vi "Scan Engine-Single Frame.vi"(7 "Channel":u32(ring)=1 items=["A"=1, "B"=2, "A + B"=3, "C"=4, "A + C"=5, "A + B"=6, "D"=8, "A + D"=9, "B + D"=10, "C + D"=12, "A + B + C + D"=15], 8 "Error in":errorcluster, 10 "Scan Status in":T1) -> (0 "Error Out":errorcluster, 2 "Buffer":u16[](array[numeric]), 3 "FFT Buffer":sgl[](array[numeric]))   [LabVIEW 2018]
uses:
  Controls/scan status.ctl
  Hardware Mfg/AlazarTech SDK/Controls/Alazar Engine Actions.ctl
  Controls/FGV Actions.ctl
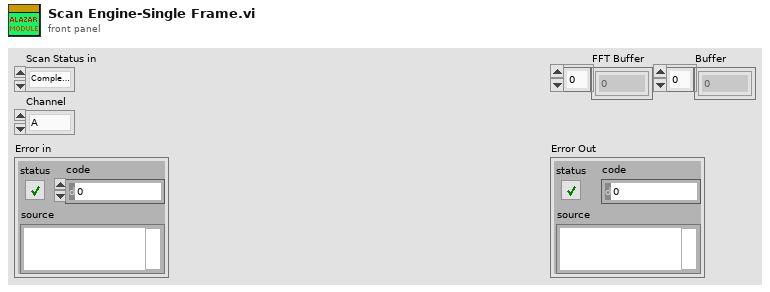
[diagram p1: front panel]
types:
  T1 = typedef "scan status.ctl" = enum16{"Complete Scan(ThorOCT)", "Complete Scan(PSOCT)", "Start(ThorOCT Spatial)", "Start(ThorOCT Spectral)", "Start(GPU FFT)", "Start(Alazar FFT)", "Scan(ThorOCT Spatial)", "Scan(ThorOCT Spectral)", "Scan(GPU FFT)", "Scan(Alazar FFT)", "Finish Scan(ThorOCT)", "Finish Scan(PSOCT)"}
  T2 = typedef "Alazar Engine Actions.ctl" = enum16{"Init", "Config Clock", "Config Ch", "Config Trig", "Config Non-FFT Acq.", "Non-FFT Acquire", "start acquire", "Config Acq.", "Acquire", "UnInit"}
  T3 = typedef "FGV Actions.ctl" = enum16{"Init", "Set", "Get", "Clear"}
  T4 = enum16{"Configure channels", "Write Scan Pattern", "Start Galvo Task", "Is Task Done?", "Stop Galvo", "Uninit", "Init: Calc scan pattern"}
  T5 = typedef "System Parameters.ctl" = cluster{"Optical Parameters":T6, "Vibratome":T7, "Table Stages":T8, "Imaging Parameter":T11, "Galvo HW Parameters":cluster{"Analog Out Channel":tag, "Min Voltage":dbl, "Max Voltage":dbl, "Pixel Clock Source":tag, "Sample Rate":dbl, "Line Clock Out Ch":tag}, "Alazar parameters":T13, "Mosaic Paramter":cluster{"X Axis":cluster{"Start [mm]":dbl, "Steps [pts]":dbl, "End [mm]":dbl}, "Y Axis":cluster{"Start [mm]":dbl, "Steps [pts]":dbl, "End [mm]":dbl}, "Scan Pattern":enum16{"Uni-directional", "Bi-Directional", "Spiral Out", "Spiral In"}, "Overlap Options":cluster{"Overlap Type":enum16{"No Overlap", "X Only", "Y Only", "X and Y"}, "Percent Overlap":u8, "Justify":enum16{"Start", "Center", "End"}}}, "Manual Controls":T20, "Vibratome Axis":T23}
  T6 = typedef "Optical Parameters.ctl" = cluster{"Obj. Focal Length [mm]":dbl, "Scan Lens EFL[mm]":dbl, "Tube Lens EFL[mm]":dbl, "Galvo V Range (+/-)":dbl, "Galvo Max Half Angle [Deg]":dbl, "Max Galvo Range[%]":dbl}
  T7 = typedef "Vibratome Parameters.ctl" = cluster{"Z Bottom [mm]":dbl, "Pre Cut Dwell [s]":dbl, "Blade Frequency [RPM]":u16, "Slice Speed [mm/s]":dbl, "Post Cut Dwell [s]":dbl, "Ramp Time [s]":dbl, "Start X [mm]":dbl, "Start Y [mm]":dbl, "Slice Length [mm]":dbl, "Slice Axis":enum16{"X Axis", "Y Axis", "Z Axis"}, "Controller VISA Ref":refnum<visa-resource-name>}
  T8 = typedef "Translation Stage Parameters.ctl" = cluster{"X Stage":T9, "Y Stage":T9, "Z Stage":T9}
  T9 = typedef "Translation Stage Cluster.ctl" = cluster{"Position":dbl, "Is.Enabled?":bool, "Is.Connected?":bool, "Device SN":string, "AccelerationMaximum":dbl, "VelocityMaximum":dbl, "Acceleration":dbl, "Velocity":dbl, "waitTimeout (ms)":i32, "Model":T10, "Is.Homed?":bool}
  T10 = typedef "Translation Stage Types.ctl" = enum16{"None", "Thorlabs LTS", "Thorlabs MLJ"}
  T11 = typedef "Imaging Parameters.ctl" = cluster{"Raster Scan Direction":T12, "Pixel Dwell Time [Clock Cycles]":u16, "Flyback Time [Clock Cycles]":u16, "XY Center [um]":cluster{"X":dbl, "Y":dbl}, "Pixel Step Size [um] X":dbl, "XY Image Size":enum16{"32 x 32", "64 x 64", "128 x 128", "256 x 256", "512 x 512", "1024 x 1024", "2048 x 2048"}, "Custom":bool, "Custom Size":cluster{"X":u16, "Y":u16}, "Line Averages":u8, "Pixel Step Size [um] Y":dbl}
  T12 = typedef "Scan Direction.ctl" = enum16{"Uni Directional", "Bi Directional", "None"}
  T13 = typedef "Alazar parameters.ctl" = cluster{"Trigger Settings":cluster{"General Trigger Settings":T14, "Trigger Engine 1":T15, "Trigger Engine 2":T15}, "Device ID":T16, "Ch A Input Control":T17, "Ch B Input Control":T17, "Acq Settings":T18, "Capture Clock":T19}
  T14 = typedef "General Trigger Settings.ctl" = cluster{"Trigger Operation":u32, "Coupling ID":u32, "Range ID":u32, "Delay":u32, "Timeout Ticks":u32, "Mode":u32, "Parameter":u32}
  T15 = typedef "Trigger Engine Controls.ctl" = cluster{"Trigger Engine":u32, "Source":u32, "Slope":u32, "Level":u32}
  T16 = typedef "Alazar Device ID.ctl" = cluster{"System ID":u32, "Board ID":u32}
  T17 = typedef "Channel Input Controls.ctl" = cluster{"Channel":u8, "Coupling":u32, "Range":u32, "Impedance":u32}
  T18 = typedef "Alazar Acquisition Settings.ctl" = cluster{"Record Length":u32, "Offset":u32, "Records Per Buffer":u32, "Records Count (Records/Acq)":u32, "Window Type":u32, "Footer":u32, "Samples per record":u32, "Output Format":u32}
  T19 = typedef "Clock Controls.ctl" = cluster{"Sample Rate":u32, "Decimation":u32, "Source":u32, "Edge":u32}
  T20 = typedef "Manual Controls.ctl" = cluster{"Z0":dbl, "First image height":dbl, "Data Path":path, "Save parameters":T21, "Center Galvos":bool, "Acquisition mode":T22, "PSOCT Channel":u32, "Save":bool, "AIP rotation angle":dbl, "Scan Parameters":cluster{"# Scan":cluster{"#Ascan":i32, "#Bscan":i32}, "# Rpt":cluster{"#ARpt":i32, "#BRpt":i32}, "Aline Rate":u16, "# Extra":cluster{"# ARpt_extra":i32, "#Brtn_extra":i32}}, "ROI Parameters":cluster{"ROI (mm)":cluster{"X (mm)":dbl, "Y (mm)":dbl}, "Shift (mm)":cluster{"Xshift (mm)":sgl, "Yshift (mm)":sgl}}, "Objective":u16}
  T21 = typedef "FFT parameters.ctl" = cluster{"start pixel":i32, "#pixels to save":i32}
  T22 = typedef "FFT mode.ctl" = enum16{"ThorOCT B line", "ThorOCT Spectral", "ThorOCT FFT", "Alazar B line", "Alazar FFT", "GPU FFT", "Alazar Spectral"}
  T23 = typedef "Vibratome Param.ctl" = cluster{"Start [mm](first cut height)":dbl, "slice thickness[um]":dbl, "#slice":u16, "slice thick2[um]":dbl, "#thin slices":u16, "image thickness(um)":dbl, "#images":u16, "image depth2":dbl, "#image depth2":u16}
  T24 = cluster{"General Trigger Settings":T14, "Trigger Engine 1":T15, "Trigger Engine 2":T15}
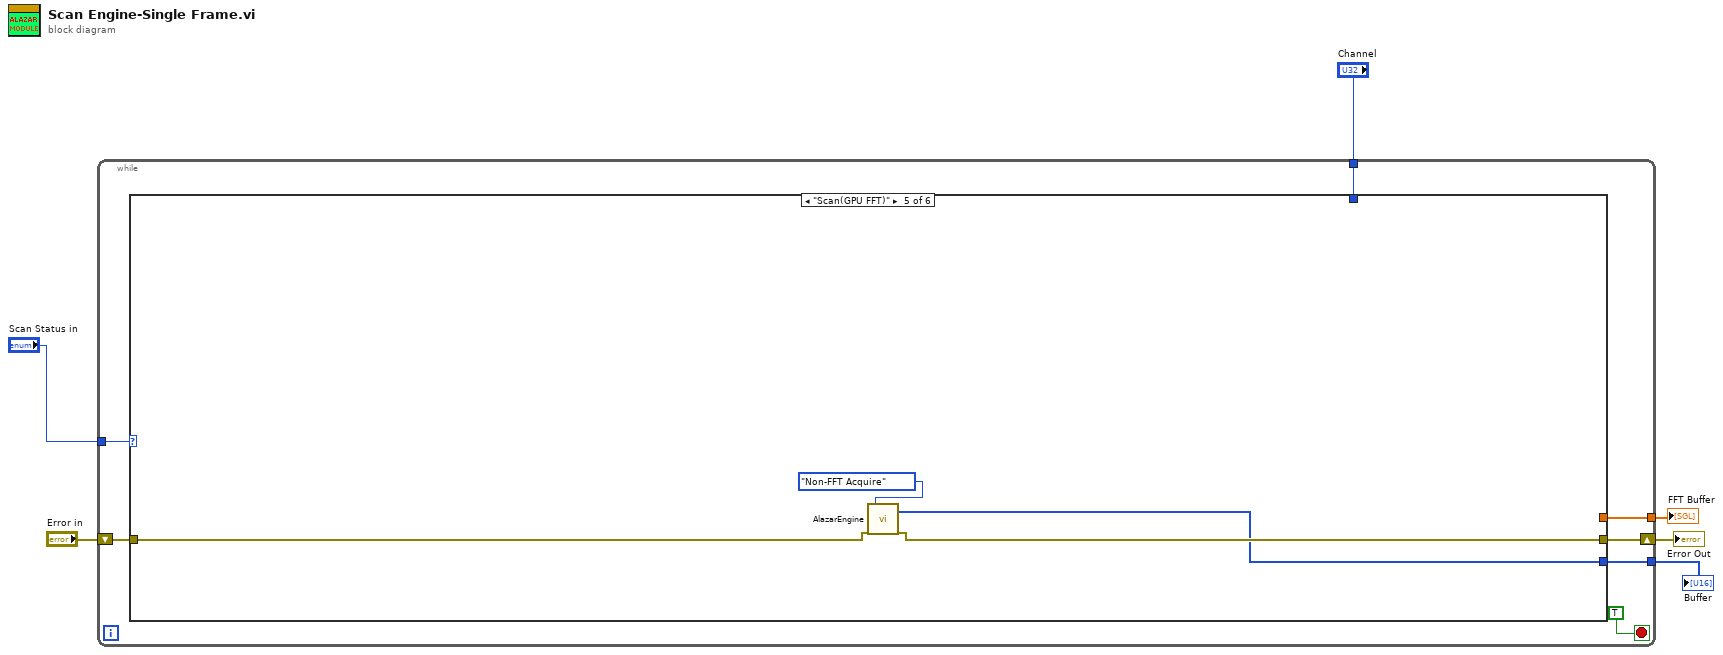
[diagram p0: block diagram]
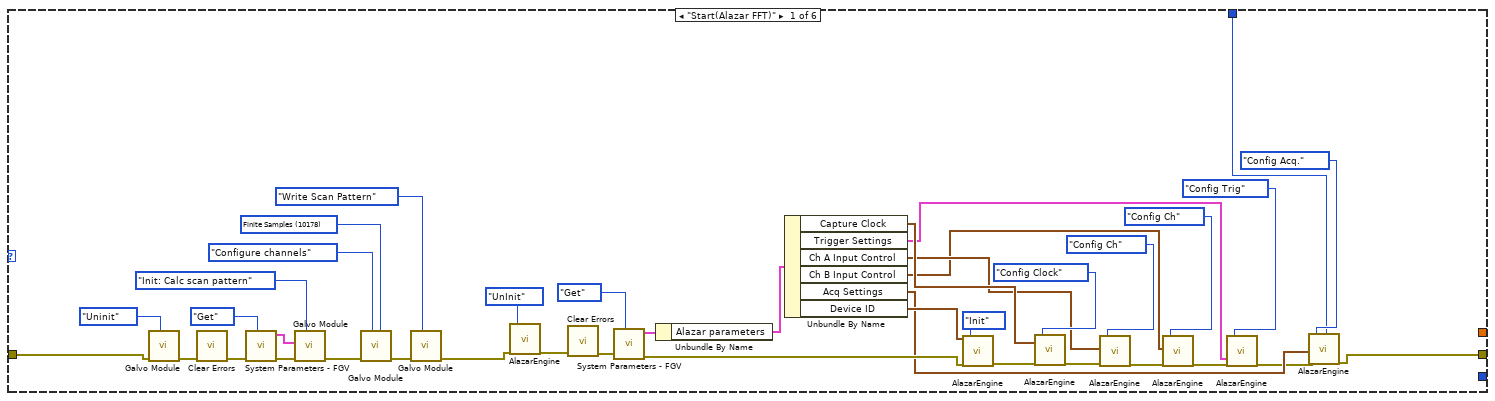
[diagram p2: hidden frame]
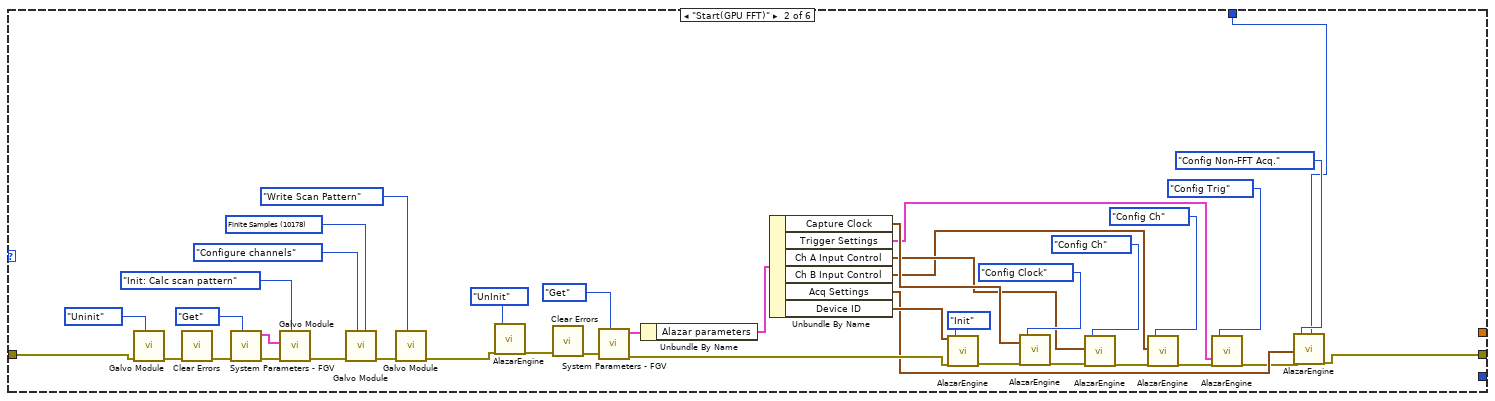
[diagram p3: hidden frame]
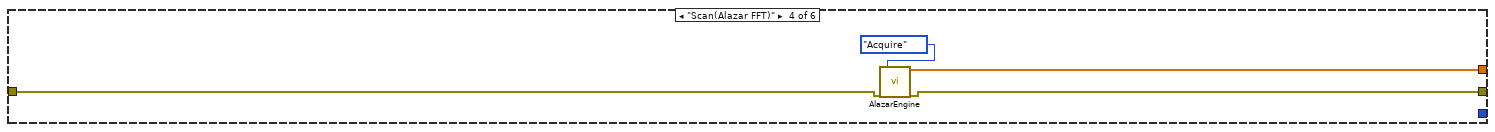
[diagram p5: hidden frame]
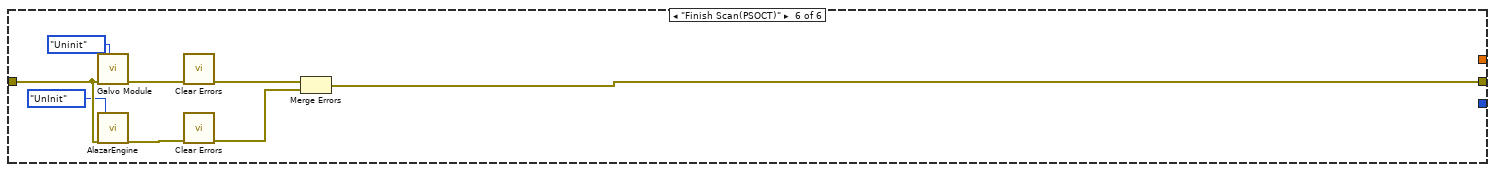
[diagram p6: hidden frame]
diagram:
  n1 = while {
    shift-right: [w12] -> w5
    shift-left: "Error in" -> [w10]
    tunnel: "Scan Status in" -> [w11]
    tunnel: [w9] -> w3
    tunnel: [w8] -> w2
    tunnel: "Channel" -> [w7]
    stop <- TRUE ("Status In") stop-if-true
    n2 = case shown="\"Scan(GPU FFT)\"" w11 {
      tunnel: w10 -> [w41 w56 w94 w97 w101 w107]
      tunnel: [w15 w55 w94 w96 w100 w104] -> w12
      tunnel: [_ _ _ w95 _ _] -> w9
      tunnel: [_ _ _ _ w99 _] -> w8
      tunnel: w7 -> [w14 w54 _ _ _ _]
      frame "Start(Alazar FFT)" {
        w50 = 10178 items=["Finite Samples"=10178, "Continuous Samples"=10123, "Hardware Timed Single Point"=12522] ("sample mode")
        n3 = call "Galvo Module.vi"("Action"=T4."Uninit", "error in (no error)"=w41) -> ("error out"=w44:errorcluster)  [unwired: 8 in, 1 out]
        n4 = call <vilib>:"Clear Errors.vi"("error in (no error)"=w44) -> ("error out"=w42:errorcluster)  [unwired: 5 in, 1 out]
        n5 = call "System Parameters - FGV.vi"("Actions"=FGV_Actions."Get", "Error In"=w42) -> ("Error Out"=w45:errorcluster, "System Parameters [Out]"=w46:T5)  [unwired: 8 in]
        n6 = call "Galvo Module.vi"("Action"=T4."Init: Calc scan pattern", "error in (no error)"=w45, "System Parameters"=w46) -> ("error out"=w52:errorcluster)  [unwired: 7 in, 1 out]
        n7 = call "Galvo Module.vi"("sample mode"=w50, "Action"=T4."Configure channels", "error in (no error)"=w52) -> ("error out"=w53:errorcluster)  [unwired: 7 in, 1 out]
        n8 = call "Galvo Module.vi"("Action"=T4."Write Scan Pattern", "error in (no error)"=w53) -> ("error out"=w36:errorcluster)  [unwired: 8 in, 1 out]
        n9 = call "AlazarEngine.vi"("error in (no error)"=w36, "Action"=Alazar_Engine_Actions."UnInit") -> ("error out"=w35:errorcluster)  [unwired: 15 in, 2 out]
        n10 = call <vilib>:"Clear Errors.vi"("error in (no error)"=w35) -> ("error out"=w37:errorcluster)  [unwired: 5 in, 1 out]
        n11 = call "System Parameters - FGV.vi"("Actions"=FGV_Actions."Get", "Error In"=w37) -> ("Error Out"=w27:errorcluster, "System Parameters [Out]"=w39:T5)  [unwired: 8 in]
        n12 = Unbundle By Name(w39) -> ("Alazar parameters"=w38:T13)
        n13 = Unbundle By Name(w38) -> ("Capture Clock"=w25:T19, "Trigger Settings"=w22:T24, "Ch A Input Control"=w24:T17, "Ch B Input Control"=w23:T17, "Acq Settings"=w21:T18, "Device ID"=w26:T16)
        n14 = call "AlazarEngine.vi"("Device ID"=w26, "error in (no error)"=w27, "Action"=Alazar_Engine_Actions."Init") -> ("error out"=w20:errorcluster)  [unwired: 14 in, 2 out]
        n15 = call "AlazarEngine.vi"("Capture Clock"=w25, "error in (no error)"=w20, "Action"=Alazar_Engine_Actions."Config Clock") -> ("error out"=w19:errorcluster)  [unwired: 14 in, 2 out]
        n16 = call "AlazarEngine.vi"("Ch Input Control"=w24, "error in (no error)"=w19, "Action"=Alazar_Engine_Actions."Config Ch") -> ("error out"=w18:errorcluster)  [unwired: 14 in, 2 out]
        n17 = call "AlazarEngine.vi"("Ch Input Control"=w23, "error in (no error)"=w18, "Action"=Alazar_Engine_Actions."Config Ch") -> ("error out"=w17:errorcluster)  [unwired: 14 in, 2 out]
        n18 = call "AlazarEngine.vi"("Trigger Settings"=w22, "error in (no error)"=w17, "Action"=Alazar_Engine_Actions."Config Trig") -> ("error out"=w16:errorcluster)  [unwired: 14 in, 2 out]
        n19 = call "AlazarEngine.vi"("Acq Settings"=w21, "error in (no error)"=w16, "Action"=Alazar_Engine_Actions."Config Acq.", "FFT Channel"=w14) -> ("error out"=w15:errorcluster)  [unwired: 13 in, 2 out]
      }
      frame "Start(GPU FFT)" {
        w90 = 10178 items=["Finite Samples"=10178, "Continuous Samples"=10123, "Hardware Timed Single Point"=12522] ("sample mode")
        n20 = call "Galvo Module.vi"("Action"=T4."Uninit", "error in (no error)"=w56) -> ("error out"=w84:errorcluster)  [unwired: 8 in, 1 out]
        n21 = call <vilib>:"Clear Errors.vi"("error in (no error)"=w84) -> ("error out"=w82:errorcluster)  [unwired: 5 in, 1 out]
        n22 = call "System Parameters - FGV.vi"("Actions"=FGV_Actions."Get", "Error In"=w82) -> ("Error Out"=w85:errorcluster, "System Parameters [Out]"=w86:T5)  [unwired: 8 in]
        n23 = call "Galvo Module.vi"("Action"=T4."Init: Calc scan pattern", "error in (no error)"=w85, "System Parameters"=w86) -> ("error out"=w92:errorcluster)  [unwired: 7 in, 1 out]
        n24 = call "Galvo Module.vi"("sample mode"=w90, "Action"=T4."Configure channels", "error in (no error)"=w92) -> ("error out"=w93:errorcluster)  [unwired: 7 in, 1 out]
        n25 = call "Galvo Module.vi"("Action"=T4."Write Scan Pattern", "error in (no error)"=w93) -> ("error out"=w77:errorcluster)  [unwired: 8 in, 1 out]
        n26 = call "AlazarEngine.vi"("error in (no error)"=w77, "Action"=Alazar_Engine_Actions."UnInit") -> ("error out"=w76:errorcluster)  [unwired: 15 in, 2 out]
        n27 = call <vilib>:"Clear Errors.vi"("error in (no error)"=w76) -> ("error out"=w78:errorcluster)  [unwired: 5 in, 1 out]
        n28 = call "System Parameters - FGV.vi"("Actions"=FGV_Actions."Get", "Error In"=w78) -> ("Error Out"=w68:errorcluster, "System Parameters [Out]"=w80:T5)  [unwired: 8 in]
        n29 = Unbundle By Name(w80) -> ("Alazar parameters"=w79:T13)
        n30 = Unbundle By Name(w79) -> ("Capture Clock"=w66:T19, "Trigger Settings"=w63:T24, "Ch A Input Control"=w65:T17, "Ch B Input Control"=w64:T17, "Acq Settings"=w62:T18, "Device ID"=w67:T16)
        n31 = call "AlazarEngine.vi"("Device ID"=w67, "error in (no error)"=w68, "Action"=Alazar_Engine_Actions."Init") -> ("error out"=w61:errorcluster)  [unwired: 14 in, 2 out]
        n32 = call "AlazarEngine.vi"("Capture Clock"=w66, "error in (no error)"=w61, "Action"=Alazar_Engine_Actions."Config Clock") -> ("error out"=w60:errorcluster)  [unwired: 14 in, 2 out]
        n33 = call "AlazarEngine.vi"("Ch Input Control"=w65, "error in (no error)"=w60, "Action"=Alazar_Engine_Actions."Config Ch") -> ("error out"=w59:errorcluster)  [unwired: 14 in, 2 out]
        n34 = call "AlazarEngine.vi"("Ch Input Control"=w64, "error in (no error)"=w59, "Action"=Alazar_Engine_Actions."Config Ch") -> ("error out"=w58:errorcluster)  [unwired: 14 in, 2 out]
        n35 = call "AlazarEngine.vi"("Trigger Settings"=w63, "error in (no error)"=w58, "Action"=Alazar_Engine_Actions."Config Trig") -> ("error out"=w57:errorcluster)  [unwired: 14 in, 2 out]
        n36 = call "AlazarEngine.vi"("Acq Settings"=w62, "error in (no error)"=w57, "Action"=Alazar_Engine_Actions."Config Non-FFT Acq.", "FFT Channel"=w54) -> ("error out"=w55:errorcluster)  [unwired: 13 in, 2 out]
      }
      frame Default {
      }
      frame "Scan(Alazar FFT)" {
        n37 = call "AlazarEngine.vi"("error in (no error)"=w97, "Action"=Alazar_Engine_Actions."Acquire") -> ("FFT Buffer"=w95:sgl[], "error out"=w96:errorcluster)  [unwired: 15 in, 1 out]
      }
      frame "Scan(GPU FFT)" {
        n38 = call "AlazarEngine.vi"("error in (no error)"=w101, "Action"=Alazar_Engine_Actions."Non-FFT Acquire") -> ("Buffer"=w99:u16[], "error out"=w100:errorcluster)  [unwired: 15 in, 1 out]
      }
      frame "Finish Scan(PSOCT)" {
        n39 = call "Galvo Module.vi"("Action"=T4."Uninit", "error in (no error)"=w107) -> ("error out"=w110:errorcluster)  [unwired: 8 in, 1 out]
        n40 = call "AlazarEngine.vi"("error in (no error)"=w107, "Action"=Alazar_Engine_Actions."UnInit") -> ("error out"=w109:errorcluster)  [unwired: 15 in, 2 out]
        n41 = call <vilib>:"Clear Errors.vi"("error in (no error)"=w110) -> ("error out"=w106:errorcluster)  [unwired: 5 in, 1 out]
        n42 = call <vilib>:"Clear Errors.vi"("error in (no error)"=w109) -> ("error out"=w105:errorcluster)  [unwired: 5 in, 1 out]
        n43 = Merge Errors(w106, w105) -> (w104:errorcluster)
      }
    }
  }
  "Error Out" <- w5
  "FFT Buffer" <- w3
  "Buffer" <- w2
